vi "Get Item Property (U16).vi"(8 "error in (no error)":errorcluster, 9 "Default Value":u16, 10 "Property Name":string, 11 "Item Ref in":T1 format="%.0x") -> (0 "error out":errorcluster, 1 "Value":u16, 3 "Item Ref out":T1 format="%.0x", 4 "Found?":bool)   [LabVIEW 2020, in "Custom Device API.lvlib"]
doc: "Returns the <B>Value</B> of a specific item <B>Property Name</B>. Properties do not inherit within a custom device, so <B>Item Ref in</B> must reference the specific item on which the property is set. \n\nFor instances with a <B>Default Value</B> input, the <B>Value</B> output returns this value if the <B>Property Name</B> is not found for the specified item. Wire data to the <B>Default Value</B> input to determine the polymorphic instance to use or manually select the instance."
uses:
  <vilib>/NI VeriStand/Custom Device API/Custom Device API.lvlib
  <vilib>/NI VeriStand/Custom Device API/Custom Device Item Ref.ctl
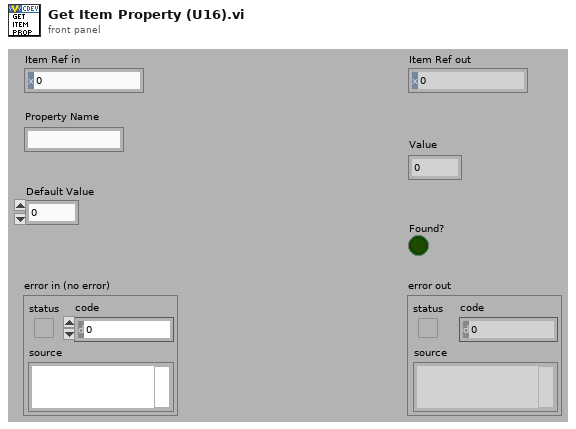
[diagram p1: front panel]
types:
  T1 = typedef "Custom Device API.lvlib/Custom Device Item Ref.ctl" = u64
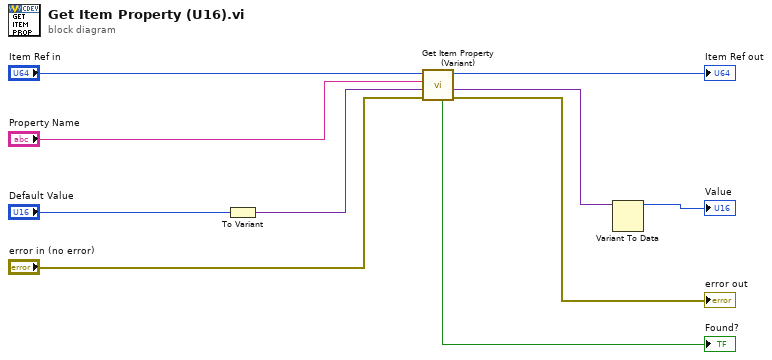
[diagram p0: block diagram]
diagram:
  n1 = To Variant(anything="Default Value") -> (Variant=w3:variant)
  n2 = call <vilib>:"Get Item Property (Variant).vi"("error in (no error)"="error in (no error)", "Default Value"=w3, "Property Name"="Property Name", "Item Ref in"="Item Ref in") -> ("error out"=→"error out":errorcluster, "Value"=w5:variant, "Item Ref out"=→"Item Ref out":T1, "Found?"=→"Found?":bool)  [unwired: 4 out]
  n3 = Variant To Data(Variant=w5) -> (data=→"Value":u16)  [unwired: 2 in, 1 out]
